vi "PH_Beckhoff_PP_PU.declare Tags.vi"(3 "error in (no error)":errorcluster, 5 "Instance Name":string) -> (0 "error out":errorcluster, 1 "PU Rack Type":T1, 2 "Data in cluster":T2={"Default Values"={"Sonderklemmen Inputs"=[], "Analog Inputs"=[], "Analog Outputs"=[], "Digital Inputs"=[], "Digital Outputs"=[]}, "Description"="", "Hardware configured?"=TRUE, "Activate Change Manager?"=FALSE, "Difference to handle an analog input as change"=1})   [LabVIEW 2014, in "PH_Beckhoff_PP_PU.lvlib"]
doc: "This VI declares the tagnames and sets the scaling of the tags of this class."
uses:
  PH_Beckhoff_PP_PU.lvlib
  PH_Beckhoff/PH_Beckhoff.constructor Data in.ctl
  PH_Beckhoff/PH_Beckhoff.Values.ctl
  PH_Beckhoff/PH_Beckhoff.Sonderklemmen Inputs.ctl
  PH_Beckhoff/PH_Beckhoff.Analog Inputs.ctl
  PH_Beckhoff/PH_Beckhoff.Scaling Type.ctl
  PH_Beckhoff/PH_Beckhoff.Analog Outputs.ctl
  PH_Beckhoff/PH_Beckhoff.Digital Inputs.ctl
  PH_Beckhoff/PH_Beckhoff.Digital Outputs.ctl
  PH_Beckhoff_PP_PU.PU Rack Type.ctl
  PH_Beckhoff/PH_Beckhoff.lvlib
  PH_Common/PH_Common.lvlib
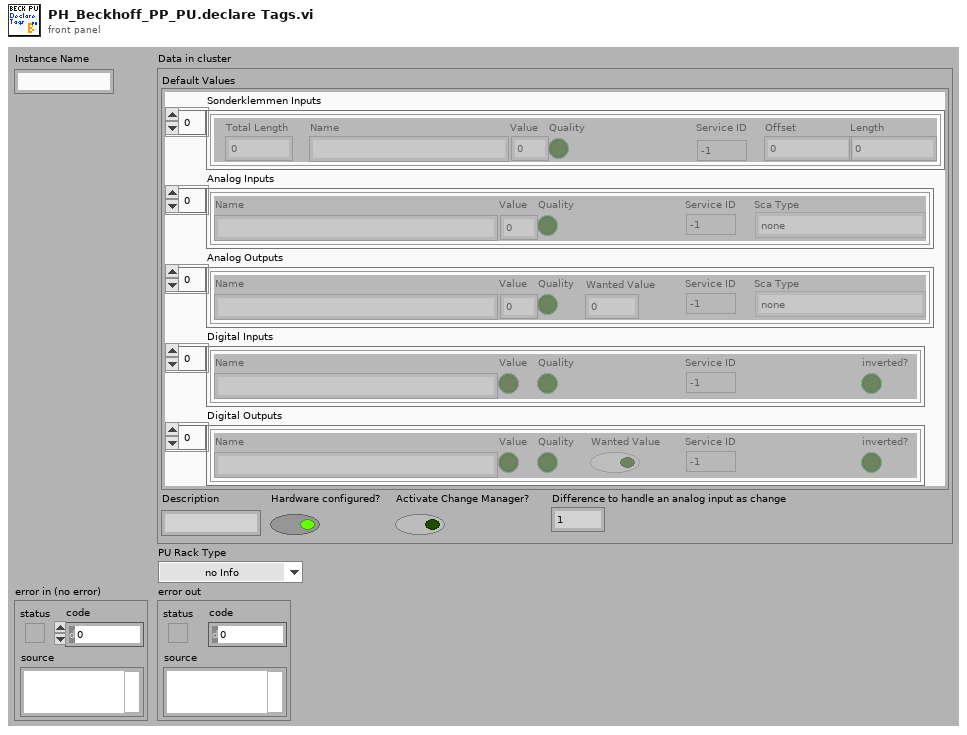
[diagram p1: front panel]
types:
  T1 = typedef "PH_Beckhoff_PP_PU.lvlib/PH_Beckhoff_PP_PU.PU Rack Type.ctl" = enum16{"no Info", "PA 19mm", "PA 45mm", "MA PU 1 and 2", "MA PU 3 and 4", "MA PU 5 and 6", "MA FR and PILC"}
  T2 = typedef "PH_Beckhoff.lvlib/PH_Beckhoff.constructor Data in.ctl" = cluster{"Default Values":T3, "Description":string, "Hardware configured?":bool, "Activate Change Manager?":bool, "Difference to handle an analog input as change":u32}
  T3 = typedef "PH_Beckhoff.lvlib/PH_Beckhoff.Values.ctl" = cluster{"Sonderklemmen Inputs":T4, "Analog Inputs":T5, "Analog Outputs":T7, "Digital Inputs":T8, "Digital Outputs":T9}
  T4 = typedef "PH_Beckhoff.lvlib/PH_Beckhoff.Sonderklemmen Inputs.ctl" = cluster{"Total Length":u32, "Name":string, "Value":u64, "Quality":bool, "Service ID":i32, "Offset":u32, "Length":u32}[]
  T5 = typedef "PH_Beckhoff.lvlib/PH_Beckhoff.Analog Inputs.ctl" = cluster{"Name":string, "Value":u32, "Quality":bool, "Service ID":i32, "Sca Type":T6}[]
  T6 = typedef "PH_Beckhoff.lvlib/PH_Beckhoff.Scaling Type.ctl" = enum16{"none", "0 ... 15 Bit -> 0 ... 5", "0 ... 15 Bit -> 0 ... 10", "0 ... 15 Bit -> 0 ... 25", "0 ... 15 Bit -> 4 ... 20", "0 ... 15 Bit -> 0 ... 1", "0 ... 15 Bit -> 0 ... 20000", "0 ... 15 Bit -> 0 ... 24000"}
  T7 = typedef "PH_Beckhoff.lvlib/PH_Beckhoff.Analog Outputs.ctl" = cluster{"Name":string, "Value":u32, "Quality":bool, "Wanted Value":u32, "Service ID":i32, "Sca Type":T6}[]
  T8 = typedef "PH_Beckhoff.lvlib/PH_Beckhoff.Digital Inputs.ctl" = cluster{"Name":string, "Value":bool, "Quality":bool, "Service ID":i32, "inverted?":bool}[]
  T9 = typedef "PH_Beckhoff.lvlib/PH_Beckhoff.Digital Outputs.ctl" = cluster{"Name":string, "Value":bool, "Quality":bool, "Wanted Value":bool, "Service ID":i32, "inverted?":bool}[]
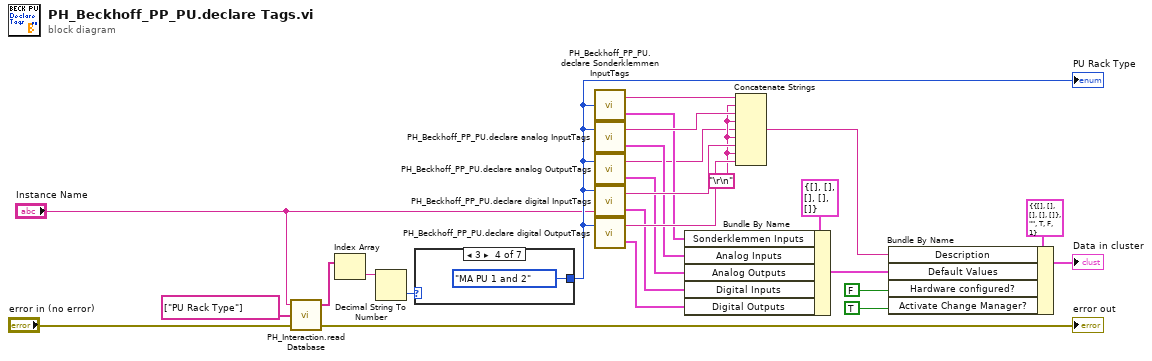
[diagram p0: block diagram]
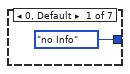
[diagram p2: hidden frame]
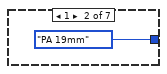
[diagram p3: hidden frame]
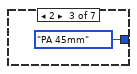
[diagram p4: hidden frame]
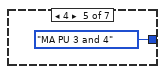
[diagram p5: hidden frame]
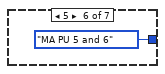
[diagram p6: hidden frame]
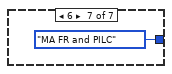
[diagram p7: hidden frame]
diagram:
  w11 = "\r\n"
  n1 = call "PH_Interaction.read Database.vi"("error in (no error)"="error in (no error)", "Strings to search for"=string[] ["PU Rack Type"] ("Strings to search for in"), "DB Entry to read"="Instance Name") -> ("error out"=→"error out":errorcluster, "Values"=w5:string[])  [unwired: 1 in]
  n2 = Index Array(array=w5) -> (element=w6:string)  [unwired: 1 in]
  n3 = Decimal String To Number(string=w6) -> (number=w4:i32)  [unwired: 2 in, 1 out]
  n4 = case shown="3" w4 {
    tunnel: [PH_Beckhoff_PP_PU.PU_Rack_Type."no Info" ("PU Type") PH_Beckhoff_PP_PU.PU_Rack_Type."PA 19mm" ("PU Type") PH_Beckhoff_PP_PU.PU_Rack_Type."PA 45mm" ("PU Type") PH_Beckhoff_PP_PU.PU_Rack_Type."MA PU 1 and 2" ("PU Type") PH_Beckhoff_PP_PU.PU_Rack_Type."MA PU 3 and 4" ("PU Type") PH_Beckhoff_PP_PU.PU_Rack_Type."MA PU 5 and 6" ("PU Type") PH_Beckhoff_PP_PU.PU_Rack_Type."MA FR and PILC" ("PU Type")] -> w3
    frame 0, Default {
    }
    frame 1 {
    }
    frame 2 {
    }
    frame 3 {
    }
    frame 4 {
    }
    frame 5 {
    }
    frame 6 {
    }
  }
  "PU Rack Type" <- w3
  n5 = call "PH_Beckhoff_PP_PU.declare Sonderklemmen InputTags.vi"("PU Type"=w3) -> ("Description"=w13:string, "Sonderklemmen Inputs"=w12:T4)
  n6 = call "PH_Beckhoff_PP_PU.declare analog InputTags.vi"("PU Type"=w3) -> ("Analog Inputs"=w17:T5, "Description"=w18:string)  [unwired: 1 in]
  n7 = call "PH_Beckhoff_PP_PU.declare analog OutputTags.vi"("PU Type"=w3) -> ("Analog Outputs"=w10:T7, "Description"=w9:string)  [unwired: 1 in]
  n8 = call "PH_Beckhoff_PP_PU.declare digital InputTags.vi"("Instance Name"="Instance Name", "PU Type"=w3) -> ("Digital Inputs"=w16:T8, "Description"=w21:string)  [unwired: 1 in]
  n9 = call "PH_Beckhoff_PP_PU.declare digital OutputTags.vi"("PU Type"=w3) -> ("Digital Outputs"=w15:T9, "Description"=w20:string)  [unwired: 1 in]
  n10 = Bundle By Name(cluster=T3 {"Sonderklemmen Inputs"=[], "Analog Inputs"=[], "Analog Outputs"=[], "Digital Inputs"=[], "Digital Outputs"=[]} ("Dummy Default Values"), "Sonderklemmen Inputs"=w12, "Analog Inputs"=w17, "Analog Outputs"=w10, "Digital Inputs"=w16, "Digital Outputs"=w15) -> (w22:T3)
  n11 = Concatenate Strings(w13, w11, w18, w11, w9, w11, w21, w11, w20) -> (w19:string)
  n12 = Bundle By Name(cluster=T2 {"Default Values"={"Sonderklemmen Inputs"=[], "Analog Inputs"=[], "Analog Outputs"=[], "Digital Inputs"=[], "Digital Outputs"=[]}, "Description"="", "Hardware configured?"=TRUE, "Activate Change Manager?"=FALSE, "Difference to handle an analog input as change"=1} ("Dummy data in cluster"), "Description"=w19, "Default Values"=w22, "Hardware configured?"=FALSE, "Activate Change Manager?"=TRUE) -> (→"Data in cluster":T2)
